vi "Intake_Case_Machine.vi"(7 "Intake_Sensor":bool, 8 "Intake_Button":bool) -> (0 "Intake_Active":bool, 1 "Arm_Defense":T2, 2 "Intake_Motor":T1, 3 "Stage_Motor":T1, 5 "Intake_Position":T3=enum."Intake Portcullis", 6 "Flipper":enum16{"Closed", "Open"}(ring)=enum."Open")   [LabVIEW 2015]
uses:
  Intake Enum..ctl
  Arm_defense_Type_Def.ctl
  Motor_Dir_Type_Def.ctl
  Intake State Type Def.ctl
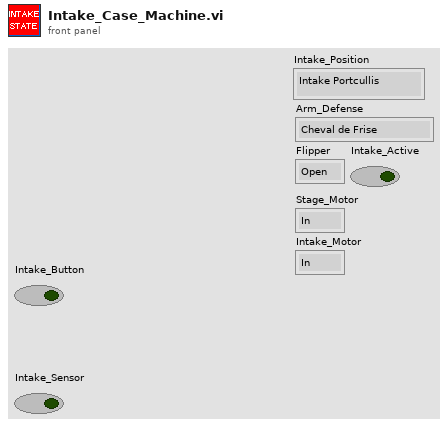
[diagram p1: front panel]
types:
  T1 = typedef "Motor_Dir_Type_Def.ctl" = enum16{"In", "Out", "Off"}
  T2 = typedef "Arm_defense_Type_Def.ctl" = enum16{"Cheval de Frise", "Portcullis", "Out", "In", "Ball_Pickup"}
  T3 = typedef "Intake Enum..ctl" = enum16{"Float", "Intake Portcullis", "Intake Ball Pickup", "Intake Cheval", " Intake Raised"}
  T4 = enum16{"Standard", "Momentary Falling", "Momentary Rising", "Momentary Falling and Rising"}
  T5 = typedef "Intake State Type Def.ctl" = enum16{"Intake Float", "Ball Stored", "Intake Lower", "Off"}
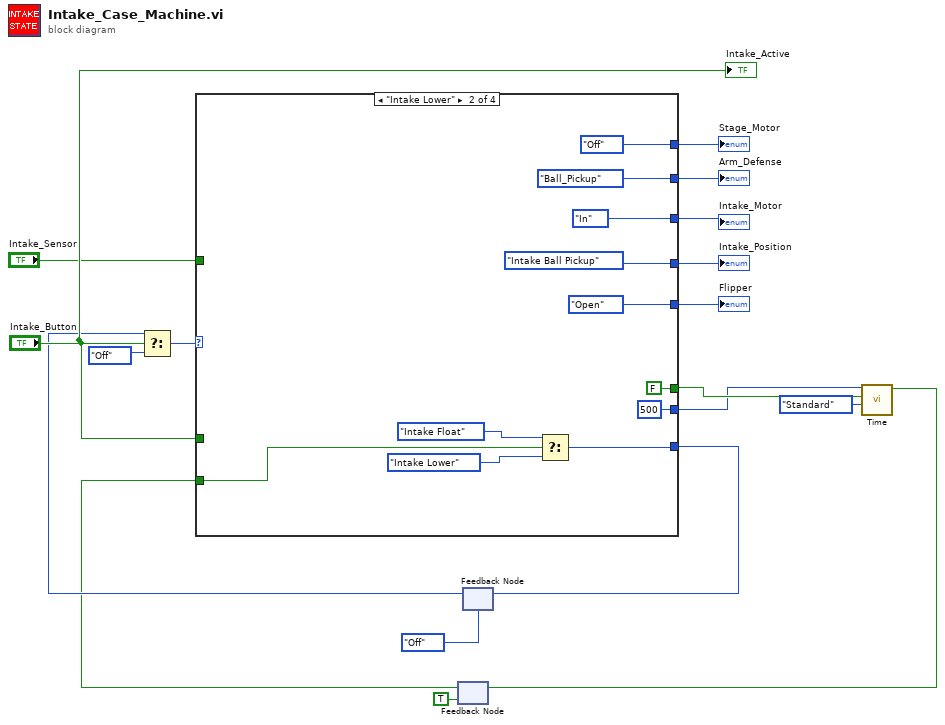
[diagram p0: block diagram]
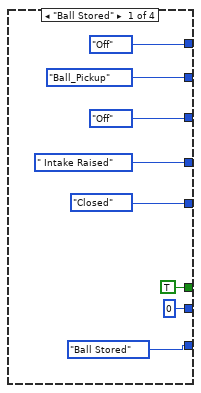
[diagram p2: hidden frame]
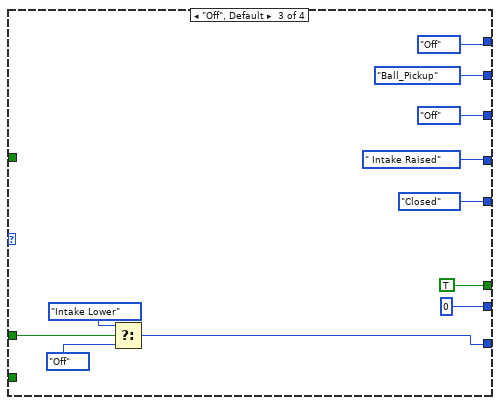
[diagram p3: hidden frame]
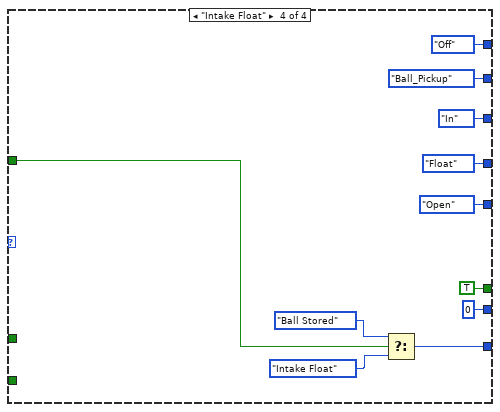
[diagram p4: hidden frame]
diagram:
  n1 = feedback #1(TRUE ("Time_Met")) -> (w4:bool)
  n2 = feedback #2(Intake_State_Type_Def."Off" ("Enum")) -> (w17:T5)
  n3 = Select(t=w17, s="Intake_Button", f=Intake_State_Type_Def."Off" ("Enum")) -> (s? t:f=w16:T5)
  n4 = case shown="\"Intake Lower\"" w16 {
    tunnel: "Intake_Button" -> [_ _ w48 _]
    tunnel: [Intake_State_Type_Def."Ball Stored" ("Enum") w37 w39 w59] -> w15
    tunnel: "Intake_Sensor" -> [_ _ _ w58]
    tunnel: [Motor_Dir_Type_Def."Off" ("Motor") Motor_Dir_Type_Def."Off" ("Motor") Motor_Dir_Type_Def."Off" ("Motor") Motor_Dir_Type_Def."Off" ("Motor")] -> w8
    tunnel: [Motor_Dir_Type_Def."Off" ("Motor") Motor_Dir_Type_Def."In" ("Motor") Motor_Dir_Type_Def."Off" ("Motor") Motor_Dir_Type_Def."In" ("Motor")] -> w7
    tunnel: [Intake_Enum.." Intake Raised" ("Enum") Intake_Enum.."Intake Ball Pickup" ("Enum") Intake_Enum.." Intake Raised" ("Enum") Intake_Enum.."Float" ("Enum")] -> w13
    tunnel: [Arm_defense_Type_Def."Ball_Pickup" ("Enum") Arm_defense_Type_Def."Ball_Pickup" ("Enum") Arm_defense_Type_Def."Ball_Pickup" ("Enum") Arm_defense_Type_Def."Ball_Pickup" ("Enum")] -> w10
    tunnel: [enum16{"Closed", "Open"}."Closed" ("Enum") enum16{"Closed", "Open"}."Open" ("Enum") enum16{"Closed", "Open"}."Closed" ("Enum") enum16{"Closed", "Open"}."Open" ("Enum")] -> w9
    tunnel: [TRUE FALSE TRUE TRUE] -> w2
    tunnel: [0 500 0 0] -> w1
    tunnel: w4 -> [_ w27 _ _]
    frame "Ball Stored" {
    }
    frame "Intake Lower" {
      n5 = Select(t=Intake_State_Type_Def."Intake Float" ("Enum"), s=w27, f=Intake_State_Type_Def."Intake Lower" ("Enum")) -> (s? t:f=w37:T5)
    }
    frame "Off", Default {
      n6 = Select(t=Intake_State_Type_Def."Intake Lower" ("Enum"), s=w48, f=Intake_State_Type_Def."Off" ("Enum")) -> (s? t:f=w39:T5)
    }
    frame "Intake Float" {
      n7 = Select(t=Intake_State_Type_Def."Ball Stored" ("Enum"), s=w58, f=Intake_State_Type_Def."Intake Float" ("Enum")) -> (s? t:f=w59:T5)
    }
  }
  "Intake_Position" <- w13
  "Arm_Defense" <- w10
  "Flipper" <- w9
  "Stage_Motor" <- w8
  "Intake_Motor" <- w7
  n8 = feedback-in #2(w15) -> ()
  n9 = call "Time.vi"("Configuration"=T4."Standard", "Reset"=w2, "Time_Limit  (ms)"=w1) -> ("Time_Met"=w5:bool)  [unwired: 8 in]
  n10 = feedback-in #1(w5) -> ()
  "Intake_Active" <- "Intake_Button"
